vi "LJT4_format_data.vi"(9 "value_array":dbl[](array[numeric]), 11 "time":timestamp) -> (3 "waveform_array_A":waveform(dbl)[](array[waveform])=[{"t0"=timestamp(0 s since 1904-01-01), "dt"=1.0, "Y"=[]}, {"t0"=timestamp(3732035173.078092 s since 1904-01-01), "dt"=1.0, "Y"=[302.8589782714844], "attributes"=variant("NI_ChannelName"=variant(string "T1"))}])   [LabVIEW 2019]
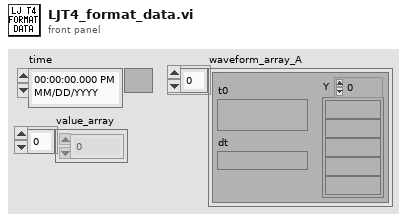
[diagram p1: front panel]
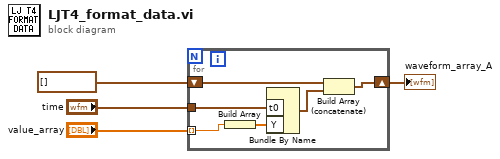
[diagram p0: block diagram]
diagram:
  n1 = for {
    tunnel: "time" -> [w8]
    tunnel: "value_array" -> [w6] mode=indexing
    shift-right: [w7] -> w4
    shift-left: waveform(dbl)[] [] -> [w10]
    n2 = Build Array(w6) -> (w9:dbl[])
    n3 = Bundle By Name("t0"=w8, "Y"=w9) -> (w5:waveform(dbl))  [unwired: 1 in]
    n4 = Build Array (concatenate)(w10, w5) -> (w7:waveform(dbl)[])
  }
  "waveform_array_A" <- w4
